vi "更换绑定设备.vi"(9 "新设备MAC":string, 10 "用户名":string, 11 "数据库连接引用.i":T1) -> (3 "数据库连接引用.o":T1)   [LabVIEW 2013, in "数据库操作.lvclass"]
uses:
  <vilib>/addons/database/Connection.llb/Conn ObjectReference.ctl
  <vilib>/addons/database/Connection.llb/Conn Execute.vi
  <vilib>/addons/database/NI_Database_API.lvlib
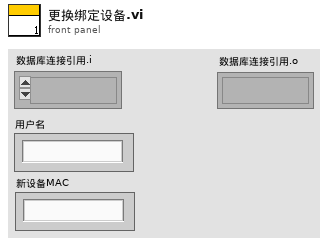
[diagram p1: front panel]
types:
  T1 = typedef "NI_Database_API.lvlib/Conn ObjectReference.ctl" = refnum<k1>
  T2 = enum16{"用户名", "设备MAC", "设备状态", "密码", "职类", "姓名", "电话", "邮箱", "备注", "最后活动"}
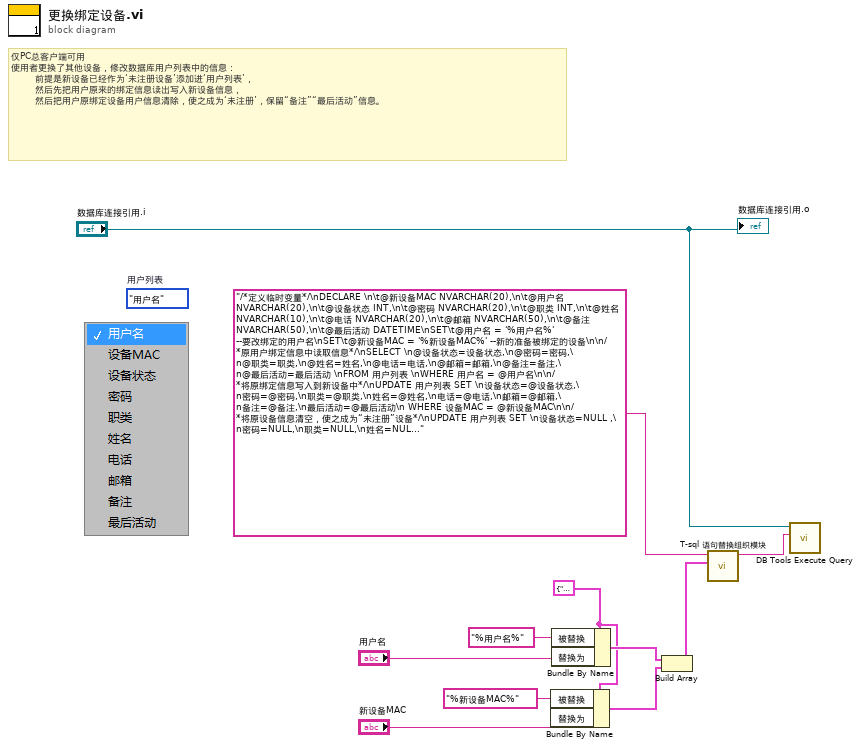
[diagram p0: block diagram]
diagram:
  w8 = cluster{"被替换":string, "替换为":string} {"被替换"="", "替换为"=""} ("替换单元")
  (unwired) T2."用户名"  # 用户列表
  # "仅PC总客户端可用\n使用者更换了其他设备，修改数据库用户列表中的信息：\n        前提是新设备已经作为‘未注册设备’添加进‘用户列表’，\n        然后先把用户原来的绑定信息读出写入新设备信息，\n        然后把用户原绑定设备用户信息清除，使之成为‘未注册’，保留“备注”“最后活动”信息。"
  n1 = Bundle By Name(cluster=w8, "被替换"="%新设备MAC%", "替换为"="新设备MAC") -> (w9:cluster{"被替换":string, "替换为":string})
  n2 = Bundle By Name(cluster=w8, "被替换"="%用户名%", "替换为"="用户名") -> (w10:cluster{"被替换":string, "替换为":string})
  n3 = Build Array(w10, w9) -> (w7:cluster{"被替换":string, "替换为":string}[])
  n4 = call "T-sql 语句替换组织模块.vi"("替换项"=w7, "T-sql 模板"="/*定义临时变量*/\nDECLARE \n\t@新设备MAC NVARCHAR(20),\n\t@用户名 NVARCHAR(20),\n\t@设备状态 INT,\n\t@密码 NVARCHAR(20),\n\t@职类 INT,\n\t@姓名 NVARCHAR(10),\n\t@电话 NVARCHAR(20),\n\t@邮箱 NVARCHAR(50),\n\t@备注 NVARCHAR(50),\n\t@最后活动 DATETIME\nSET\t@用户名 = '%用户名%'  --要改绑定的用户名\nSET\t@新设备MAC = '%新设备MAC%' --新的准备被绑定的设备\n\n/*原用户绑定信息中读取信息*/\nSELECT \n@设备状态=设备状态,\n@密码=密码,\n@职类=职类,\n@姓名=姓名,\n@电话=电话,\n@邮箱=邮箱,\n@备注=备注,\n@最后活动=最后活动 \nFROM 用户列表 \nWHERE 用户名 = @用户名\n\n/*将原绑定信息写入到新设备中*/\nUPDATE 用户列表 SET \n设备状态=@设备状态,\n密码=@密码,\n职类=@职类,\n姓名=@姓名,\n电话=@电话,\n邮箱=@邮箱,\n备注=@备注,\n最后活动=@最后活动\n WHERE 设备MAC = @新设备MAC\n\n/*将原设备信息清空，使之成为“未注册”设备*/\nUPDATE 用户列表 SET \n设备状态=NULL ,\n密码=NULL,\n职类=NULL,\n姓名=NULL,\n电话=NULL,\n邮箱=NULL \nWHERE 设备MAC = @新设备MAC AND 用户名 <> @用户名\n") -> ("T-sql"=w2:string)  [unwired: 8 in, 1 out]
  n5 = call-poly <vilib>:"DB Tools Execute Query.vi"("SQL query"=w2, "connection reference"="数据库连接引用.i") -> ()  [unwired: 6 in, 2 out]
  "数据库连接引用.o" <- "数据库连接引用.i"
